vi "detElementName.vi"(8 "error in (no error)":errorcluster, 10 "XML In":string, 11 "Element in":refnum<class "XMLParser.lvclass">) -> (0 "error out":errorcluster, 3 "Element out":refnum<class "XMLParser.lvclass">)   [LabVIEW 2014, in "XML.lvlib" / "XMLParser.lvclass"]
doc: "This method determines the XML element name from the XML input string."
uses:
  <userlib>/Common/XML/XMLParser/XMLParser.lvclass
  <userlib>/Common/XML/XMLParser/XMLParser.lvclass/XMLParser.ctl
  <vilib>/Utility/error.llb/Trim Whitespace.vi
  <userlib>/Common/XML/XMLAttributeParser/XMLAttributeParser.lvclass
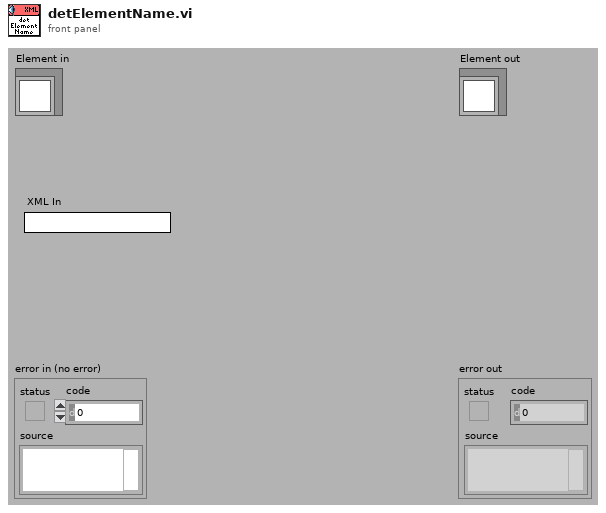
[diagram p1: front panel]
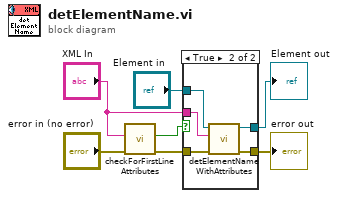
[diagram p0: block diagram]
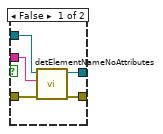
[diagram p2: hidden frame]
diagram:
  n1 = call <userlib>:"checkForFirstLineAttributes.vi"("error in (no error)"="error in (no error)", "XML In"="XML In") -> ("error out"=w1:errorcluster, "firstLineAttributeFound"=w3:bool)  [unwired: 7 in, 1 out]
  n2 = case shown="True" w3 {
    tunnel: "XML In" -> [w12 w15]
    tunnel: w1 -> [w9 w17]
    tunnel: [w8 w16] -> w7
    tunnel: "Element in" -> [w11 w13]
    tunnel: [w10 w14] -> w5
    frame False {
      n3 = call <userlib>:"detElementNameNoAttributes.vi"("error in (no error)"=w9, "XML In"=w12, "ReadElement Out"=w11) -> ("error out"=w8:errorcluster, "ReadElement Out"=w10:refnum<class "XMLParser.lvclass">)  [unwired: 6 in, 1 out]
    }
    frame True {
      n4 = call <userlib>:"detElementNameWithAttributes.vi"("error in (no error)"=w17, "XML In"=w15, "Element in"=w13) -> ("error out"=w16:errorcluster, "Element out"=w14:refnum<class "XMLParser.lvclass">)  [unwired: 6 in, 1 out]
    }
  }
  "error out" <- w7
  "Element out" <- w5
